vi "PicoScope6000aExampleRapidBlockBulk.vi"() -> ()   [LabVIEW 2009]
uses:
  <vilib>/Waveform/DWDTOps.llb/DWDT Analog to Digital.vi
panel:
  in  "Channels":T1 {"Channel H Settings"."Range" items=["10mV", "20mV", "50mV", "100mV", "200mV", "500mV", "1V", "2V", "5V", "10V", "20V", "50V", "100V", "200V", "x10_Probe_100mV", "x10_Probe_200mV", "x10_Probe_500mV", "x10_Probe_1V", "x10_Probe_2V", "x10_Probe_5V", "x10_Probe_10V", "x10_Probe_20V", "x10_Probe_50V", "x10_Probe_100V", "x10_Probe_200V", "x10_Probe_500V", "CURRENT_CLAMP_60A_2A", "CURRENT_CLAMP_60A_5A", "CURRENT_CLAMP_60A_10A", "CURRENT_CLAMP_60A_20A", "CURRENT_CLAMP_60A_50A", "CURRENT_CLAMP_60A_60A", "CURRENT_CLAMP_60A_V2_0_5A", "CURRENT_CLAMP_60A_V2_1A", "CURRENT_CLAMP_60A_V2_2A", "CURRENT_CLAMP_60A_V2_5A", "CURRENT_CLAMP_60A_V2_10A", "CURRENT_CLAMP_60A_V2_20A", "CURRENT_CLAMP_60A_V2_50A", "CURRENT_CLAMP_60A_V2_60A", "RESISTANCE_LEAD_NEG5_TO_20OHM", "RESISTANCE_LEAD_NEG50_TO_200OHM", "RESISTANCE_LEAD_NEG500_TO_2KOHM", "RESISTANCE_LEAD_NEG5K_TO_20KOHM", "RESISTANCE_LEAD_NEG50K_TO_LEAD_200KOHM", "RESISTANCE_LEAD_NEG500K_TO_LEAD_2MOHM", "RESISTANCE_LEAD_DIODE_TEST", "HT_NEG3_TO_5KV", "HT_NEG3_TO_10KV", "HT_NEG5_TO_20KV", "HT_NEG5_TO_50KV", "HT_NEG5_TO_100KV", "HT_NEG3_TO_5KV_INVERTED", "HT_NEG3_TO_10KV_INVERTED", "HT_NEG5_TO_20KV_INVERTED", "HT_NEG5_TO_50KV_INVERTED", "HT_NEG5_TO_100KV_INVERTED", "TEMPERATURE_NEG50_TO_150DEGC", "PRESSURE_SENSOR_-100k-150k_PASCALS", "PRESSURE_SENSOR_-100k_TO_400k_PASCALS", "PRESSURE_SENSOR_-200k_TO_800k_PASCALS", "PRESSURE_SENSOR_-400k_TO_1600k_PASCALS", "PRESSURE_SENSOR_-400k_TO_3400k_PASCALS", "PRESSURE_SENSOR_-150k_TO_1350k_PASCALS"]; "Channel H Settings"."BandWidth" items=["Full", "100kHz", "20kHz", "1MHz", "20MHz", "25MHz", "50MHz", "250MHz", "500MHz"]; "Channel H Settings"."Coupling" items=["AC", "DC"]; "Channel G Settings"."Range" items=["10mV", "20mV", "50mV", "100mV", "200mV", "500mV", "1V", "2V", "5V", "10V", "20V", "50V", "100V", "200V", "x10_Probe_100mV", "x10_Probe_200mV", "x10_Probe_500mV", "x10_Probe_1V", "x10_Probe_2V", "x10_Probe_5V", "x10_Probe_10V", "x10_Probe_20V", "x10_Probe_50V", "x10_Probe_100V", "x10_Probe_200V", "x10_Probe_500V", "CURRENT_CLAMP_60A_2A", "CURRENT_CLAMP_60A_5A", "CURRENT_CLAMP_60A_10A", "CURRENT_CLAMP_60A_20A", "CURRENT_CLAMP_60A_50A", "CURRENT_CLAMP_60A_60A", "CURRENT_CLAMP_60A_V2_0_5A", "CURRENT_CLAMP_60A_V2_1A", "CURRENT_CLAMP_60A_V2_2A", "CURRENT_CLAMP_60A_V2_5A", "CURRENT_CLAMP_60A_V2_10A", "CURRENT_CLAMP_60A_V2_20A", "CURRENT_CLAMP_60A_V2_50A", "CURRENT_CLAMP_60A_V2_60A", "RESISTANCE_LEAD_NEG5_TO_20OHM", "RESISTANCE_LEAD_NEG50_TO_200OHM", "RESISTANCE_LEAD_NEG500_TO_2KOHM", "RESISTANCE_LEAD_NEG5K_TO_20KOHM", "RESISTANCE_LEAD_NEG50K_TO_LEAD_200KOHM", "RESISTANCE_LEAD_NEG500K_TO_LEAD_2MOHM", "RESISTANCE_LEAD_DIODE_TEST", "HT_NEG3_TO_5KV", "HT_NEG3_TO_10KV", "HT_NEG5_TO_20KV", "HT_NEG5_TO_50KV", "HT_NEG5_TO_100KV", "HT_NEG3_TO_5KV_INVERTED", "HT_NEG3_TO_10KV_INVERTED", "HT_NEG5_TO_20KV_INVERTED", "HT_NEG5_TO_50KV_INVERTED", "HT_NEG5_TO_100KV_INVERTED", "TEMPERATURE_NEG50_TO_150DEGC", "PRESSURE_SENSOR_-100k-150k_PASCALS", "PRESSURE_SENSOR_-100k_TO_400k_PASCALS", "PRESSURE_SENSOR_-200k_TO_800k_PASCALS", "PRESSURE_SENSOR_-400k_TO_1600k_PASCALS", "PRESSURE_SENSOR_-400k_TO_3400k_PASCALS", "PRESSURE_SENSOR_-150k_TO_1350k_PASCALS"]; "Channel G Settings"."BandWidth" items=["Full", "100kHz", "20kHz", "1MHz", "20MHz", "25MHz", "50MHz", "250MHz", "500MHz"]; "Channel G Settings"."Coupling" items=["AC", "DC"]; "Channel F Settings"."Range" items=["10mV", "20mV", "50mV", "100mV", "200mV", "500mV", "1V", "2V", "5V", "10V", "20V", "50V", "100V", "200V", "x10_Probe_100mV", "x10_Probe_200mV", "x10_Probe_500mV", "x10_Probe_1V", "x10_Probe_2V", "x10_Probe_5V", "x10_Probe_10V", "x10_Probe_20V", "x10_Probe_50V", "x10_Probe_100V", "x10_Probe_200V", "x10_Probe_500V", "CURRENT_CLAMP_60A_2A", "CURRENT_CLAMP_60A_5A", "CURRENT_CLAMP_60A_10A", "CURRENT_CLAMP_60A_20A", "CURRENT_CLAMP_60A_50A", "CURRENT_CLAMP_60A_60A", "CURRENT_CLAMP_60A_V2_0_5A", "CURRENT_CLAMP_60A_V2_1A", "CURRENT_CLAMP_60A_V2_2A", "CURRENT_CLAMP_60A_V2_5A", "CURRENT_CLAMP_60A_V2_10A", "CURRENT_CLAMP_60A_V2_20A", "CURRENT_CLAMP_60A_V2_50A", "CURRENT_CLAMP_60A_V2_60A", "RESISTANCE_LEAD_NEG5_TO_20OHM", "RESISTANCE_LEAD_NEG50_TO_200OHM", "RESISTANCE_LEAD_NEG500_TO_2KOHM", "RESISTANCE_LEAD_NEG5K_TO_20KOHM", "RESISTANCE_LEAD_NEG50K_TO_LEAD_200KOHM", "RESISTANCE_LEAD_NEG500K_TO_LEAD_2MOHM", "RESISTANCE_LEAD_DIODE_TEST", "HT_NEG3_TO_5KV", "HT_NEG3_TO_10KV", "HT_NEG5_TO_20KV", "HT_NEG5_TO_50KV", "HT_NEG5_TO_100KV", "HT_NEG3_TO_5KV_INVERTED", "HT_NEG3_TO_10KV_INVERTED", "HT_NEG5_TO_20KV_INVERTED", "HT_NEG5_TO_50KV_INVERTED", "HT_NEG5_TO_100KV_INVERTED", "TEMPERATURE_NEG50_TO_150DEGC", "PRESSURE_SENSOR_-100k-150k_PASCALS", "PRESSURE_SENSOR_-100k_TO_400k_PASCALS", "PRESSURE_SENSOR_-200k_TO_800k_PASCALS", "PRESSURE_SENSOR_-400k_TO_1600k_PASCALS", "PRESSURE_SENSOR_-400k_TO_3400k_PASCALS", "PRESSURE_SENSOR_-150k_TO_1350k_PASCALS"]; "Channel F Settings"."BandWidth" items=["Full", "100kHz", "20kHz", "1MHz", "20MHz", "25MHz", "50MHz", "250MHz", "500MHz"]; "Channel F Settings"."Coupling" items=["AC", "DC"]; "Channel E Settings"."Range" items=["10mV", "20mV", "50mV", "100mV", "200mV", "500mV", "1V", "2V", "5V", "10V", "20V", "50V", "100V", "200V", "x10_Probe_100mV", "x10_Probe_200mV", "x10_Probe_500mV", "x10_Probe_1V", "x10_Probe_2V", "x10_Probe_5V", "x10_Probe_10V", "x10_Probe_20V", "x10_Probe_50V", "x10_Probe_100V", "x10_Probe_200V", "x10_Probe_500V", "CURRENT_CLAMP_60A_2A", "CURRENT_CLAMP_60A_5A", "CURRENT_CLAMP_60A_10A", "CURRENT_CLAMP_60A_20A", "CURRENT_CLAMP_60A_50A", "CURRENT_CLAMP_60A_60A", "CURRENT_CLAMP_60A_V2_0_5A", "CURRENT_CLAMP_60A_V2_1A", "CURRENT_CLAMP_60A_V2_2A", "CURRENT_CLAMP_60A_V2_5A", "CURRENT_CLAMP_60A_V2_10A", "CURRENT_CLAMP_60A_V2_20A", "CURRENT_CLAMP_60A_V2_50A", "CURRENT_CLAMP_60A_V2_60A", "RESISTANCE_LEAD_NEG5_TO_20OHM", "RESISTANCE_LEAD_NEG50_TO_200OHM", "RESISTANCE_LEAD_NEG500_TO_2KOHM", "RESISTANCE_LEAD_NEG5K_TO_20KOHM", "RESISTANCE_LEAD_NEG50K_TO_LEAD_200KOHM", "RESISTANCE_LEAD_NEG500K_TO_LEAD_2MOHM", "RESISTANCE_LEAD_DIODE_TEST", "HT_NEG3_TO_5KV", "HT_NEG3_TO_10KV", "HT_NEG5_TO_20KV", "HT_NEG5_TO_50KV", "HT_NEG5_TO_100KV", "HT_NEG3_TO_5KV_INVERTED", "HT_NEG3_TO_10KV_INVERTED", "HT_NEG5_TO_20KV_INVERTED", "HT_NEG5_TO_50KV_INVERTED", "HT_NEG5_TO_100KV_INVERTED", "TEMPERATURE_NEG50_TO_150DEGC", "PRESSURE_SENSOR_-100k-150k_PASCALS", "PRESSURE_SENSOR_-100k_TO_400k_PASCALS", "PRESSURE_SENSOR_-200k_TO_800k_PASCALS", "PRESSURE_SENSOR_-400k_TO_1600k_PASCALS", "PRESSURE_SENSOR_-400k_TO_3400k_PASCALS", "PRESSURE_SENSOR_-150k_TO_1350k_PASCALS"]; "Channel E Settings"."BandWidth" items=["Full", "100kHz", "20kHz", "1MHz", "20MHz", "25MHz", "50MHz", "250MHz", "500MHz"]; "Channel E Settings"."Coupling" items=["AC", "DC"]; "Channel D Settings"."Range" items=["10mV", "20mV", "50mV", "100mV", "200mV", "500mV", "1V", "2V", "5V", "10V", "20V", "50V", "100V", "200V", "x10_Probe_100mV", "x10_Probe_200mV", "x10_Probe_500mV", "x10_Probe_1V", "x10_Probe_2V", "x10_Probe_5V", "x10_Probe_10V", "x10_Probe_20V", "x10_Probe_50V", "x10_Probe_100V", "x10_Probe_200V", "x10_Probe_500V", "CURRENT_CLAMP_60A_2A", "CURRENT_CLAMP_60A_5A", "CURRENT_CLAMP_60A_10A", "CURRENT_CLAMP_60A_20A", "CURRENT_CLAMP_60A_50A", "CURRENT_CLAMP_60A_60A", "CURRENT_CLAMP_60A_V2_0_5A", "CURRENT_CLAMP_60A_V2_1A", "CURRENT_CLAMP_60A_V2_2A", "CURRENT_CLAMP_60A_V2_5A", "CURRENT_CLAMP_60A_V2_10A", "CURRENT_CLAMP_60A_V2_20A", "CURRENT_CLAMP_60A_V2_50A", "CURRENT_CLAMP_60A_V2_60A", "RESISTANCE_LEAD_NEG5_TO_20OHM", "RESISTANCE_LEAD_NEG50_TO_200OHM", "RESISTANCE_LEAD_NEG500_TO_2KOHM", "RESISTANCE_LEAD_NEG5K_TO_20KOHM", "RESISTANCE_LEAD_NEG50K_TO_LEAD_200KOHM", "RESISTANCE_LEAD_NEG500K_TO_LEAD_2MOHM", "RESISTANCE_LEAD_DIODE_TEST", "HT_NEG3_TO_5KV", "HT_NEG3_TO_10KV", "HT_NEG5_TO_20KV", "HT_NEG5_TO_50KV", "HT_NEG5_TO_100KV", "HT_NEG3_TO_5KV_INVERTED", "HT_NEG3_TO_10KV_INVERTED", "HT_NEG5_TO_20KV_INVERTED", "HT_NEG5_TO_50KV_INVERTED", "HT_NEG5_TO_100KV_INVERTED", "TEMPERATURE_NEG50_TO_150DEGC", "PRESSURE_SENSOR_-100k-150k_PASCALS", "PRESSURE_SENSOR_-100k_TO_400k_PASCALS", "PRESSURE_SENSOR_-200k_TO_800k_PASCALS", "PRESSURE_SENSOR_-400k_TO_1600k_PASCALS", "PRESSURE_SENSOR_-400k_TO_3400k_PASCALS", "PRESSURE_SENSOR_-150k_TO_1350k_PASCALS"]; "Channel D Settings"."BandWidth" items=["Full", "100kHz", "20kHz", "1MHz", "20MHz", "25MHz", "50MHz", "250MHz", "500MHz"]; "Channel D Settings"."Coupling" items=["AC", "DC"]; "Channel C Settings"."Range" items=["10mV", "20mV", "50mV", "100mV", "200mV", "500mV", "1V", "2V", "5V", "10V", "20V", "50V", "100V", "200V", "x10_Probe_100mV", "x10_Probe_200mV", "x10_Probe_500mV", "x10_Probe_1V", "x10_Probe_2V", "x10_Probe_5V", "x10_Probe_10V", "x10_Probe_20V", "x10_Probe_50V", "x10_Probe_100V", "x10_Probe_200V", "x10_Probe_500V", "CURRENT_CLAMP_60A_2A", "CURRENT_CLAMP_60A_5A", "CURRENT_CLAMP_60A_10A", "CURRENT_CLAMP_60A_20A", "CURRENT_CLAMP_60A_50A", "CURRENT_CLAMP_60A_60A", "CURRENT_CLAMP_60A_V2_0_5A", "CURRENT_CLAMP_60A_V2_1A", "CURRENT_CLAMP_60A_V2_2A", "CURRENT_CLAMP_60A_V2_5A", "CURRENT_CLAMP_60A_V2_10A", "CURRENT_CLAMP_60A_V2_20A", "CURRENT_CLAMP_60A_V2_50A", "CURRENT_CLAMP_60A_V2_60A", "RESISTANCE_LEAD_NEG5_TO_20OHM", "RESISTANCE_LEAD_NEG50_TO_200OHM", "RESISTANCE_LEAD_NEG500_TO_2KOHM", "RESISTANCE_LEAD_NEG5K_TO_20KOHM", "RESISTANCE_LEAD_NEG50K_TO_LEAD_200KOHM", "RESISTANCE_LEAD_NEG500K_TO_LEAD_2MOHM", "RESISTANCE_LEAD_DIODE_TEST", "HT_NEG3_TO_5KV", "HT_NEG3_TO_10KV", "HT_NEG5_TO_20KV", "HT_NEG5_TO_50KV", "HT_NEG5_TO_100KV", "HT_NEG3_TO_5KV_INVERTED", "HT_NEG3_TO_10KV_INVERTED", "HT_NEG5_TO_20KV_INVERTED", "HT_NEG5_TO_50KV_INVERTED", "HT_NEG5_TO_100KV_INVERTED", "TEMPERATURE_NEG50_TO_150DEGC", "PRESSURE_SENSOR_-100k-150k_PASCALS", "PRESSURE_SENSOR_-100k_TO_400k_PASCALS", "PRESSURE_SENSOR_-200k_TO_800k_PASCALS", "PRESSURE_SENSOR_-400k_TO_1600k_PASCALS", "PRESSURE_SENSOR_-400k_TO_3400k_PASCALS", "PRESSURE_SENSOR_-150k_TO_1350k_PASCALS"]; "Channel C Settings"."BandWidth" items=["Full", "100kHz", "20kHz", "1MHz", "20MHz", "25MHz", "50MHz", "250MHz", "500MHz"]; "Channel C Settings"."Coupling" items=["AC", "DC"]; "Channel B Settings"."Range" items=["10mV", "20mV", "50mV", "100mV", "200mV", "500mV", "1V", "2V", "5V", "10V", "20V", "50V", "100V", "200V", "x10_Probe_100mV", "x10_Probe_200mV", "x10_Probe_500mV", "x10_Probe_1V", "x10_Probe_2V", "x10_Probe_5V", "x10_Probe_10V", "x10_Probe_20V", "x10_Probe_50V", "x10_Probe_100V", "x10_Probe_200V", "x10_Probe_500V", "CURRENT_CLAMP_60A_2A", "CURRENT_CLAMP_60A_5A", "CURRENT_CLAMP_60A_10A", "CURRENT_CLAMP_60A_20A", "CURRENT_CLAMP_60A_50A", "CURRENT_CLAMP_60A_60A", "CURRENT_CLAMP_60A_V2_0_5A", "CURRENT_CLAMP_60A_V2_1A", "CURRENT_CLAMP_60A_V2_2A", "CURRENT_CLAMP_60A_V2_5A", "CURRENT_CLAMP_60A_V2_10A", "CURRENT_CLAMP_60A_V2_20A", "CURRENT_CLAMP_60A_V2_50A", "CURRENT_CLAMP_60A_V2_60A", "RESISTANCE_LEAD_NEG5_TO_20OHM", "RESISTANCE_LEAD_NEG50_TO_200OHM", "RESISTANCE_LEAD_NEG500_TO_2KOHM", "RESISTANCE_LEAD_NEG5K_TO_20KOHM", "RESISTANCE_LEAD_NEG50K_TO_LEAD_200KOHM", "RESISTANCE_LEAD_NEG500K_TO_LEAD_2MOHM", "RESISTANCE_LEAD_DIODE_TEST", "HT_NEG3_TO_5KV", "HT_NEG3_TO_10KV", "HT_NEG5_TO_20KV", "HT_NEG5_TO_50KV", "HT_NEG5_TO_100KV", "HT_NEG3_TO_5KV_INVERTED", "HT_NEG3_TO_10KV_INVERTED", "HT_NEG5_TO_20KV_INVERTED", "HT_NEG5_TO_50KV_INVERTED", "HT_NEG5_TO_100KV_INVERTED", "TEMPERATURE_NEG50_TO_150DEGC", "PRESSURE_SENSOR_-100k-150k_PASCALS", "PRESSURE_SENSOR_-100k_TO_400k_PASCALS", "PRESSURE_SENSOR_-200k_TO_800k_PASCALS", "PRESSURE_SENSOR_-400k_TO_1600k_PASCALS", "PRESSURE_SENSOR_-400k_TO_3400k_PASCALS", "PRESSURE_SENSOR_-150k_TO_1350k_PASCALS"]; "Channel B Settings"."BandWidth" items=["Full", "100kHz", "20kHz", "1MHz", "20MHz", "25MHz", "50MHz", "250MHz", "500MHz"]; "Channel B Settings"."Coupling" items=["AC", "DC"]; "Channel A Settings"."Range" items=["10mV", "20mV", "50mV", "100mV", "200mV", "500mV", "1V", "2V", "5V", "10V", "20V", "50V", "100V", "200V", "x10_Probe_100mV", "x10_Probe_200mV", "x10_Probe_500mV", "x10_Probe_1V", "x10_Probe_2V", "x10_Probe_5V", "x10_Probe_10V", "x10_Probe_20V", "x10_Probe_50V", "x10_Probe_100V", "x10_Probe_200V", "x10_Probe_500V", "CURRENT_CLAMP_60A_2A", "CURRENT_CLAMP_60A_5A", "CURRENT_CLAMP_60A_10A", "CURRENT_CLAMP_60A_20A", "CURRENT_CLAMP_60A_50A", "CURRENT_CLAMP_60A_60A", "CURRENT_CLAMP_60A_V2_0_5A", "CURRENT_CLAMP_60A_V2_1A", "CURRENT_CLAMP_60A_V2_2A", "CURRENT_CLAMP_60A_V2_5A", "CURRENT_CLAMP_60A_V2_10A", "CURRENT_CLAMP_60A_V2_20A", "CURRENT_CLAMP_60A_V2_50A", "CURRENT_CLAMP_60A_V2_60A", "RESISTANCE_LEAD_NEG5_TO_20OHM", "RESISTANCE_LEAD_NEG50_TO_200OHM", "RESISTANCE_LEAD_NEG500_TO_2KOHM", "RESISTANCE_LEAD_NEG5K_TO_20KOHM", "RESISTANCE_LEAD_NEG50K_TO_LEAD_200KOHM", "RESISTANCE_LEAD_NEG500K_TO_LEAD_2MOHM", "RESISTANCE_LEAD_DIODE_TEST", "HT_NEG3_TO_5KV", "HT_NEG3_TO_10KV", "HT_NEG5_TO_20KV", "HT_NEG5_TO_50KV", "HT_NEG5_TO_100KV", "HT_NEG3_TO_5KV_INVERTED", "HT_NEG3_TO_10KV_INVERTED", "HT_NEG5_TO_20KV_INVERTED", "HT_NEG5_TO_50KV_INVERTED", "HT_NEG5_TO_100KV_INVERTED", "TEMPERATURE_NEG50_TO_150DEGC", "PRESSURE_SENSOR_-100k-150k_PASCALS", "PRESSURE_SENSOR_-100k_TO_400k_PASCALS", "PRESSURE_SENSOR_-200k_TO_800k_PASCALS", "PRESSURE_SENSOR_-400k_TO_1600k_PASCALS", "PRESSURE_SENSOR_-400k_TO_3400k_PASCALS", "PRESSURE_SENSOR_-150k_TO_1350k_PASCALS"]; "Channel A Settings"."BandWidth" items=["Full", "100kHz", "20kHz", "1MHz", "20MHz", "25MHz", "50MHz", "250MHz", "500MHz"]; "Channel A Settings"."Coupling" items=["AC", "DC"]}
  out "overflow":i16[](array[numeric]) format="%08b"
  out "nMaxSamples":u64
  in  "Buffer and Transfer Settings":T2 {"Down-Sample Mode" items=["None", "Aggregate", "Decimate", "Average"]; "Down Sample Ratio" step=1; "noOfSamples" format="%#_6p"}
  in  "Acquisition Settings":T3 {"postTriggerSamples" format="%#_6p"; "preTriggerSamples" format="%#_6p"}
  out "Capture Complete":bool
  out "Number of Samples \nPer Capture":u64 format="%#_6p"
  in  "Run":bool
  in  "Capture Index":i16 min=0
  in  "Digital Channels":T4 {"Port 1 Settings"."Hysteresis" items=["PICO_VERY_HIGH_400MV", "PICO_HIGH_200MV", "PICO_NORMAL_100MV", "PICO_LOW_50MV"]; "Port 0 Settings"."Hysteresis" items=["PICO_VERY_HIGH_400MV", "PICO_HIGH_200MV", "PICO_NORMAL_100MV", "PICO_LOW_50MV"]}
  out "Properties Panel":T5 {"Max Total Capture Time Available (sec)" format="%.3p"; "Sample Frequency" format="%.6p"; "Sample Rate" format="%.3p"; "Max Samples Available" format="%_6p"; "Total Capture Time (sec)" format="%.3p"}
  out "Port 0":digitalwaveform(graph)
  in  "Trigger Settings":T6 {"Trigger Source" items=["Channel A", "Channel B", "Channel C", "Channel D", "Channel E", "Channel F", "Channel G", "Channel H", "Port 0", "Port 1", "Trigger AUX"]; "Trigger Direction" items=["Rising", "Falling"]; "Trigger Threshold (Volts)" format="%#_6p"}
  in  "stop":bool
  out "Analog Channels":cluster{i32, dbl, "Data (Volts)":dbl[]}[](graph)
  out "Device Info":T7
  out "Pico 6000a Units":string
  in  "Resolution":u32(ring) items=["8-bit", "12-bit", "14-bit", "15-bit", "16-bit", "10-bit"]
  in  "Serial Number":string
  in  "Use Serial Number":bool
  in  "error in (no error)":errorcluster
  # "Please Ensure you set the \"Range\"(Probe type) before running the VI"
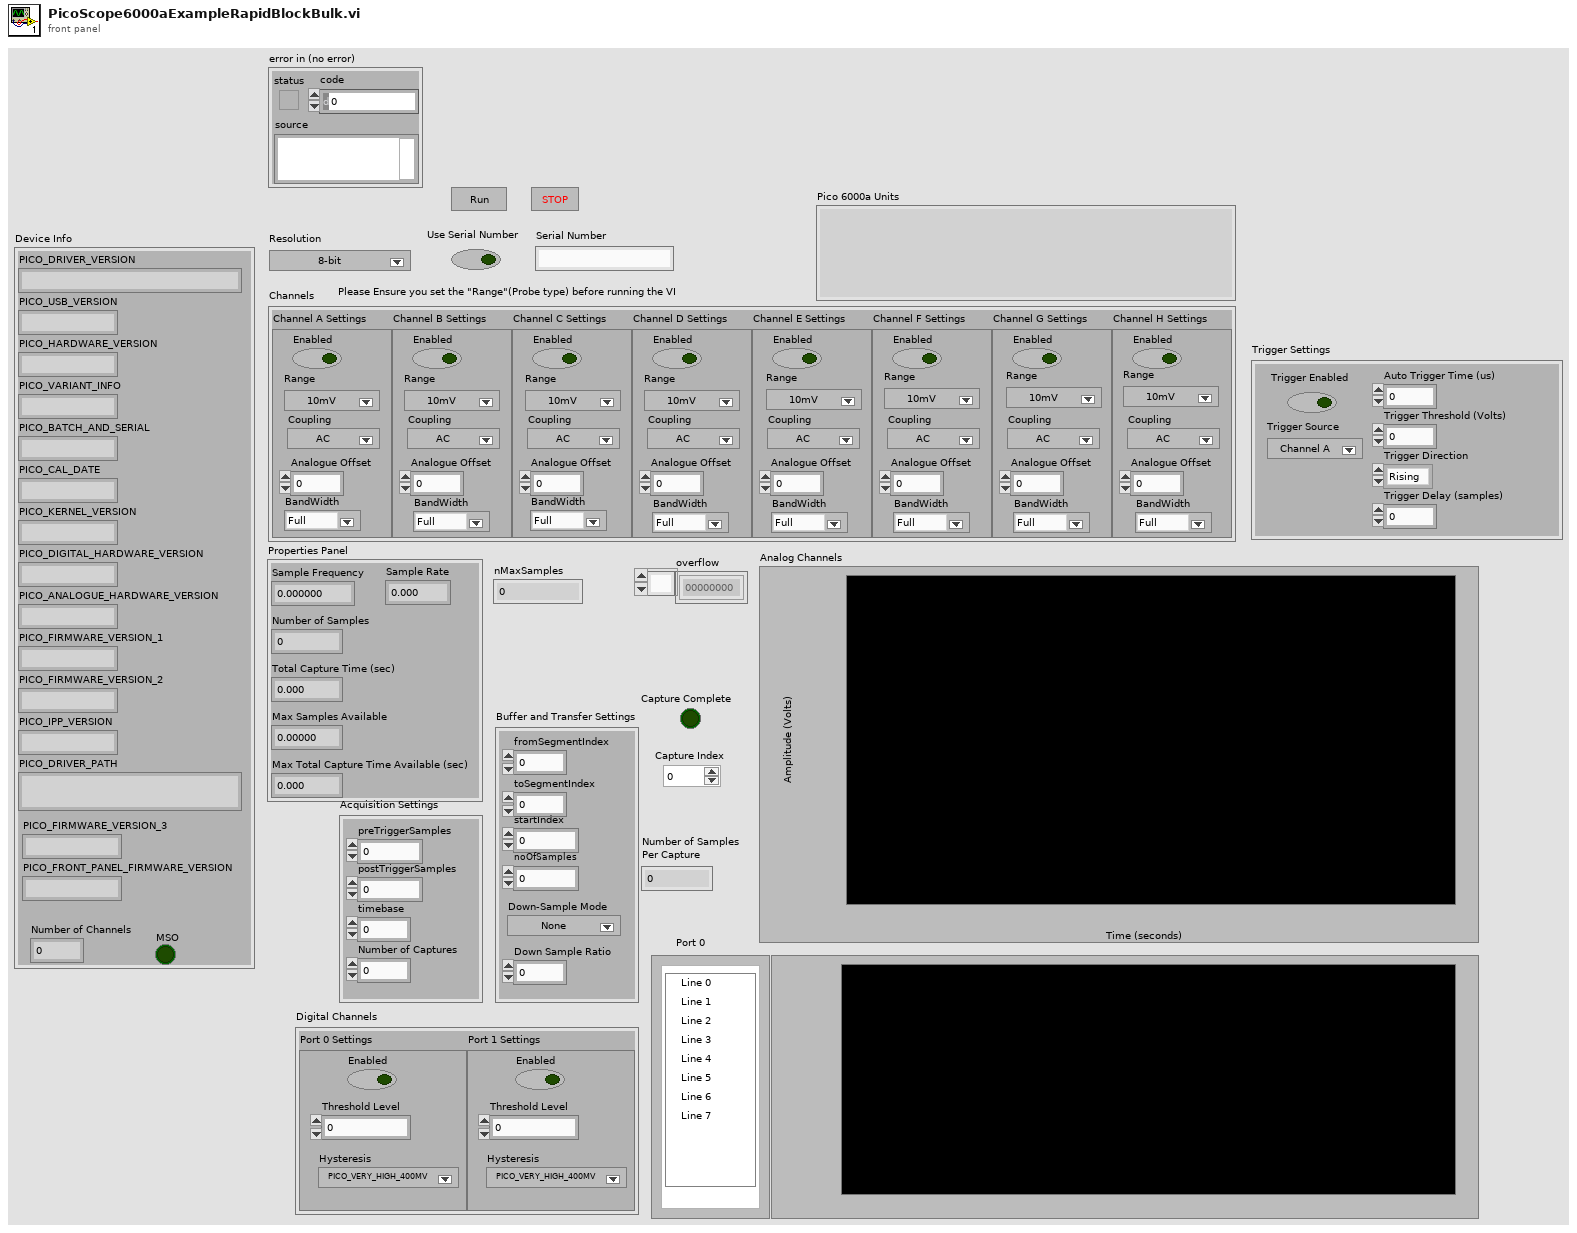
[diagram p1: front panel]
types:
  T1 = cluster{"Channel A Settings ":cluster{"Enabled":bool, "Coupling":i16, "Range":u16, "Analogue Offset":dbl, "BandWidth":u32}, "Channel B Settings ":cluster{"Enabled":bool, "Coupling":i16, "Range":u16, "Analogue Offset":dbl, "BandWidth":u32}, "Channel C Settings ":cluster{"Enabled":bool, "Coupling":i16, "Range":u16, "Analogue Offset":dbl, "BandWidth":u32}, "Channel D Settings ":cluster{"Enabled":bool, "Coupling":i16, "Range":u16, "Analogue Offset":dbl, "BandWidth":u32}, "Channel E Settings":cluster{"Enabled":bool, "Coupling":i16, "Range":u16, "Analogue Offset":dbl, "BandWidth":u32}, "Channel F Settings":cluster{"Enabled":bool, "Coupling":i16, "Range":u16, "Analogue Offset":dbl, "BandWidth":u32}, "Channel G Settings":cluster{"Enabled":bool, "Coupling":i16, "Range":u16, "Analogue Offset":dbl, "BandWidth":u32}, "Channel H Settings ":cluster{"Enabled":bool, "Coupling":i16, "Range":u16, "Analogue Offset":dbl, "BandWidth":u32}}
  T2 = cluster{"fromSegmentIndex":u64, "toSegmentIndex":u64, "startIndex":u64, "noOfSamples":u64, "Down-Sample Mode":u32, "Down Sample Ratio":u64}
  T3 = cluster{"preTriggerSamples":u64, "postTriggerSamples":u64, "timebase":u32, "Number of Captures":u64}
  T4 = cluster{"Port 0 Settings ":cluster{"Enabled":bool, "Threshold Level":i16, "Hysteresis":u32}, "Port 1 Settings":cluster{"Enabled":bool, "Threshold Level":i16, "Hysteresis":u32}}
  T5 = cluster{"Sample Frequency":dbl, "Sample Rate":dbl, "Max Samples Available":u64, "Number of Samples":u64, "Total Capture Time (sec) ":dbl, "Max Total Capture Time Available (sec)":dbl}
  T6 = cluster{"Trigger Enabled":bool, "Trigger Threshold (Volts)":dbl, "Trigger Direction":u16, "Trigger Delay (samples)":u64, "Auto Trigger Time (us)":u32, "Trigger Source":u32}
  T7 = cluster{"PICO_DRIVER_VERSION":string, "PICO_USB_VERSION":string, "PICO_HARDWARE_VERSION":string, "PICO_VARIANT_INFO":string, "PICO_BATCH_AND_SERIAL":string, "PICO_CAL_DATE":string, "PICO_KERNEL_VERSION":string, "PICO_DIGITAL_HARDWARE_VERSION":string, "PICO_ANALOGUE_HARDWARE_VERSION":string, "PICO_FIRMWARE_VERSION_1":string, "PICO_FIRMWARE_VERSION_2":string, "PICO_IPP_VERSION":string, "PICO_DRIVER_PATH":string, "PICO_FIRMWARE_VERSION_3":string, "PICO_FRONT_PANEL_FIRMWARE_VERSION":string, "Number of Channels":i16, "MSO":bool}
  T8 = cluster{"bufferMax ChA":i16[][], "bufferMax ChB":i16[][], "bufferMax ChC":i16[][], "bufferMax ChD":i16[][], "bufferMax ChE":i16[][], "bufferMin ChF":i16[][], "bufferMin ChG":i16[][], "bufferMax ChH":i16[][], "bufferMax Port0":i16[][], "bufferMax Port1":i16[][]}
  T9 = cluster{"preTriggerSamples":u64, "postTriggerSamples":u64, "timebase":u32}
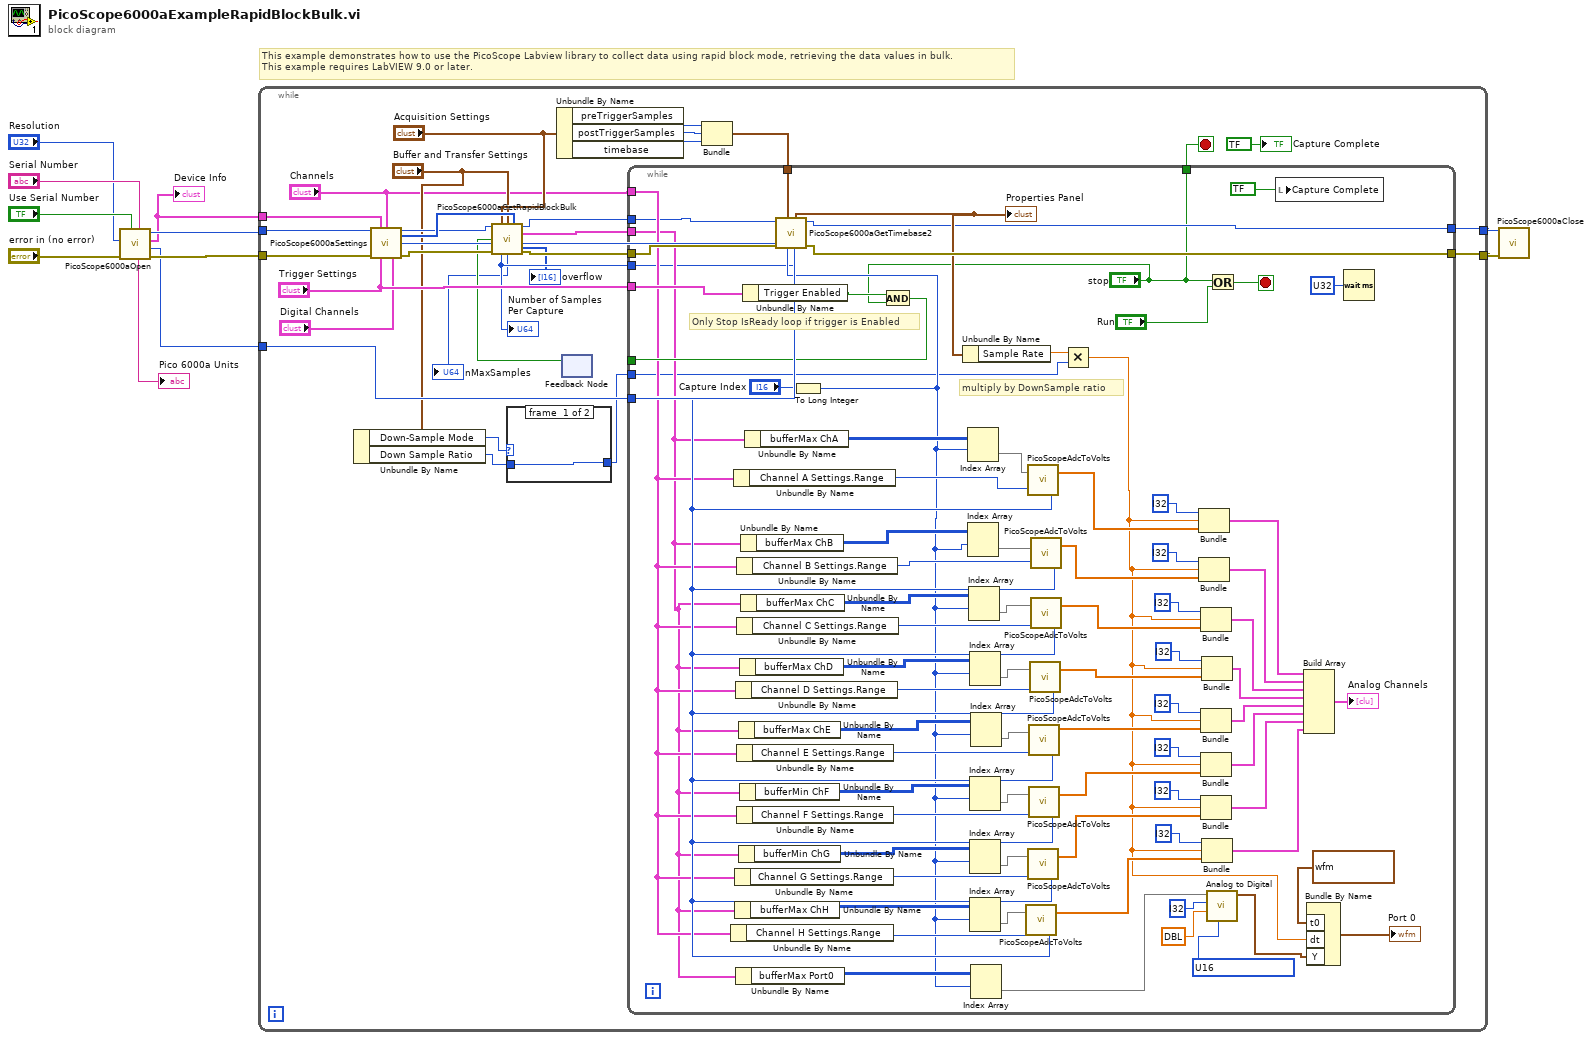
[diagram p0: block diagram]
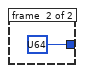
[diagram p2: hidden frame]
diagram:
  # "This example demonstrates how to use the PicoScope Labview library to collect data using rapid block mode, retrieving the data values in bulk.\nThis example requires LabVIEW 9.0 or later."
  n1 = call "PicoScope6000aOpen.vi"("Serial Number"="Serial Number", "Use Serial Number"="Use Serial Number", "error in (no error)"="error in (no error)", "Resolution"="Resolution") -> ("error out"=w7:errorcluster, "Max ADC value"=w1:i16, "Device Info"=w2:T7, "handle out"=w8:i16, "Pico 6000a Units"=→"Pico 6000a Units":string)  [unwired: 2 in, 1 out]
  "Device Info" <- w2
  n2 = while {
    tunnel: w2 -> [w40]
    tunnel: w1 -> [w37]
    tunnel: w8 -> [w42]
    tunnel: [w34] -> w6
    tunnel: w7 -> [w41]
    tunnel: [w35] -> w5
    stop <- w30 stop-if-true
    n3 = Unbundle By Name("Buffer and Transfer Settings") -> ("Down-Sample Mode"=w17:u32, "Down Sample Ratio"=w16:u64)
    n4 = call "PicoScope6000aSettings.vi"("handle in"=w42, "Device Info"=w40, "Channels"="Channels", "Max ADC value"=w37, "error in (no error)"=w41, "Trigger Settings"="Trigger Settings", "Digital Channels"="Digital Channels") -> ("Enabled array"=w39:i16[], "handle out"=w27:i16, "error out"=w29:errorcluster)  [unwired: 6 in]
    n5 = case shown="80000000" w17 {
      tunnel: [w43 u64 ? ("Down Sample Ratio")] -> w15
      tunnel: w16 -> [w43 _]
      frame #0 {
      }
      frame #1 {
      }
    }
    n6 = Unbundle By Name("Acquisition Settings") -> ("preTriggerSamples"=w23:u64, "postTriggerSamples"=w22:u64, "timebase"=w21:u32)
    n7 = feedback #1() -> (w24:bool)  [unwired: 1 in]
    n8 = call "PicoScope6000aGetRapidBlockBulk.vi"("handle in"=w27, "Acquisition Settings"="Acquisition Settings", "Buffer and Transfer Settings"="Buffer and Transfer Settings", "enabled array"=w39, "stop IsReady"=w24, "error in (no error)"=w29) -> ("handle out"=w26:i16, "Buffers (Max or non-aggregated)"=w33:T8, "noOfSamples"=w32:u64, "nMaxSamples"=→"nMaxSamples":u64, "overflow"=→"overflow":i16[], "error out"=w28:errorcluster)  [unwired: 3 in, 1 out]
    "Number of Samples \nPer Capture" <- w32
    n9 = Bundle("preTriggerSamples"=w23, "postTriggerSamples"=w22, "timebase"=w21) -> (w20:T9)  [unwired: 1 in]
    n10 = while {
      tunnel: "Trigger Settings" -> [w85]
      tunnel: w37 -> [w83]
      tunnel: [w82] -> w25
      tunnel: "Channels" -> [w72]
      tunnel: w33 -> [w62]
      tunnel: w32 -> [w60]
      tunnel: [w75] -> w34
      tunnel: w26 -> [w57]
      tunnel: w28 -> [w78]
      tunnel: [w77] -> w35
      tunnel: ["stop"] -> w30
      tunnel: w20 -> [w54]
      tunnel: w15 -> [w45]
      stop <- w56 stop-if-true
      w90 = u16 ? items=["unsigned binary", "offset binary", "2's complement"] ("data format (offset binary)")
      # "multiply by DownSample ratio"
      # "Only Stop IsReady loop if trigger is Enabled"
      n11 = Unbundle By Name(w72) -> ("Channel H Settings.Range"=w110:u16)
      n12 = Unbundle By Name(w72) -> ("Channel A Settings.Range"=w123:u16)
      n13 = Unbundle By Name(w72) -> ("Channel G Settings.Range"=w111:u16)
      n14 = Unbundle By Name(w62) -> ("bufferMax ChH"=w69:i16[][])
      n15 = Unbundle By Name(w72) -> ("Channel D Settings.Range"=w114:u16)
      n16 = Unbundle By Name(w62) -> ("bufferMax Port0"=w73:i16[][])
      n17 = Unbundle By Name(w72) -> ("Channel B Settings.Range"=w121:u16)
      n18 = Unbundle By Name(w72) -> ("Channel C Settings.Range"=w115:u16)
      n19 = Unbundle By Name(w72) -> ("Channel E Settings.Range"=w113:u16)
      n20 = Unbundle By Name(w72) -> ("Channel F Settings.Range"=w112:u16)
      n21 = Unbundle By Name(w62) -> ("bufferMax ChE"=w66:i16[][])
      n22 = Unbundle By Name(w62) -> ("bufferMin ChG"=w68:i16[][])
      n23 = Unbundle By Name(w62) -> ("bufferMax ChD"=w65:i16[][])
      n24 = Unbundle By Name(w62) -> ("bufferMin ChF"=w67:i16[][])
      n25 = Unbundle By Name(w62) -> ("bufferMax ChB"=w70:i16[][])
      n26 = Unbundle By Name(w62) -> ("bufferMax ChC"=w64:i16[][])
      n27 = Unbundle By Name(w85) -> ("Trigger Enabled"=w84:bool)
      n28 = Unbundle By Name(w62) -> ("bufferMax ChA"=w80:i16[][])
      n29 = To Long Integer(number="Capture Index") -> (32bit integer=w63:i32)
      n30 = call "PicoScope6000aGetTimebase2.vi"("Number of Samples"=w60, "Memory Segment"=w63, "Acquisition Settings"=w54, "error in (no error)"=w78, "handle in"=w57) -> ("error out"=w77:errorcluster, "handle out"=w75:i16, "Properties Panel"=w76:T5)  [unwired: 4 in]
      "Properties Panel" <- w76
      n31 = And(x=w84, y="stop") -> (x .and. y?=w82:bool)
      n32 = Unbundle By Name(w76) -> ("Sample Rate"=w46:dbl)
      n33 = Index Array(array=w80, index (row)=w63) -> (element=w79:i16[])  [unwired: 1 in]
      n34 = Index Array(array=w70, index (row)=w63) -> (element=w71:i16[])  [unwired: 1 in]
      n35 = Index Array(array=w64, index (row)=w63) -> (element=w53:i16[])  [unwired: 1 in]
      n36 = Index Array(array=w65, index (row)=w63) -> (element=w52:i16[])  [unwired: 1 in]
      n37 = Index Array(array=w67, index (row)=w63) -> (element=w50:i16[])  [unwired: 1 in]
      n38 = Index Array(array=w68, index (row)=w63) -> (element=w49:i16[])  [unwired: 1 in]
      n39 = Index Array(array=w69, index (row)=w63) -> (element=w48:i16[])  [unwired: 1 in]
      n40 = Index Array(array=w66, index (row)=w63) -> (element=w51:i16[])  [unwired: 1 in]
      n41 = Index Array(array=w73, index (row)=w63) -> (element=w74:i16[])  [unwired: 1 in]
      n42 = call "PicoScopeAdcToVolts.vi"("Max_adc"=w83, "Range Index"=w110, "Data"=w48) -> ("Data (Volts)"=w105:dbl[])
      n43 = call "PicoScopeAdcToVolts.vi"("Max_adc"=w83, "Range Index"=w123, "Data"=w79) -> ("Data (Volts)"=w120:dbl[])
      n44 = call "PicoScopeAdcToVolts.vi"("Max_adc"=w83, "Range Index"=w111, "Data"=w49) -> ("Data (Volts)"=w99:dbl[])
      n45 = call "PicoScopeAdcToVolts.vi"("Max_adc"=w83, "Range Index"=w113, "Data"=w51) -> ("Data (Volts)"=w102:dbl[])
      n46 = call "PicoScopeAdcToVolts.vi"("Max_adc"=w83, "Range Index"=w112, "Data"=w50) -> ("Data (Volts)"=w98:dbl[])
      n47 = call "PicoScopeAdcToVolts.vi"("Max_adc"=w83, "Range Index"=w114, "Data"=w52) -> ("Data (Volts)"=w103:dbl[])
      n48 = call "PicoScopeAdcToVolts.vi"("Max_adc"=w83, "Range Index"=w121, "Data"=w71) -> ("Data (Volts)"=w119:dbl[])
      n49 = call "PicoScopeAdcToVolts.vi"("Max_adc"=w83, "Range Index"=w115, "Data"=w53) -> ("Data (Volts)"=w104:dbl[])
      n50 = Multiply(x=w46, y=w45) -> (x*y=w47:dbl)
      n51 = Bundle(i32 ?, w47, "Data (Volts)"=w120) -> (w118:cluster{i32, dbl, "Data (Volts)":dbl[]})  [unwired: 1 in]
      n52 = Bundle(i32 ?, w47, "Data (Volts)"=w119) -> (w117:cluster{i32, dbl, "Data (Volts)":dbl[]})  [unwired: 1 in]
      n53 = Bundle(i32 ?, w47, "Data (Volts)"=w104) -> (w97:cluster{i32, dbl, "Data (Volts)":dbl[]})  [unwired: 1 in]
      n54 = Bundle(i32 ?, w47, "Data (Volts)"=w102) -> (w95:cluster{i32, dbl, "Data (Volts)":dbl[]})  [unwired: 1 in]
      n55 = Bundle(i32 ?, w47, "Data (Volts)"=w98) -> (w94:cluster{i32, dbl, "Data (Volts)":dbl[]})  [unwired: 1 in]
      n56 = Bundle(i32 ?, w47, "Data (Volts)"=w99) -> (w93:cluster{i32, dbl, "Data (Volts)":dbl[]})  [unwired: 1 in]
      n57 = Bundle(i32 ?, w47, "Data (Volts)"=w103) -> (w96:cluster{i32, dbl, "Data (Volts)":dbl[]})  [unwired: 1 in]
      n58 = Bundle(i32 ?, w47, "Data (Volts)"=w105) -> (w92:cluster{i32, dbl, "Data (Volts)":dbl[]})  [unwired: 1 in]
      n59 = call-poly <vilib>:"Analog to Digital.vi"("data format (offset binary)"=w90, "full-scale range (pk-pk)"=dbl ?, "resolution (16 bit)"=i32 ?, "analog waveform"=w74) -> ("digital waveform"=w86:digitalwaveform)  [unwired: 4 in, 3 out]
      n60 = Or(x="stop", y="Run") -> (x .or. y?=w56:bool)
      n61 = local write "Capture Complete"(bool ? ("Capture Complete")) -> ()
      n62 = Build Array(w118, w117, w97, w96, w95, w94, w93, w92) -> (→"Analog Channels":cluster{i32, dbl, "Data (Volts)":dbl[]}[])
      n63 = Bundle By Name("t0"=timestamp ?, "dt"=w47, "Y"=w86) -> (→"Port 0":digitalwaveform)  [unwired: 1 in]
      n64 = Wait (ms)(milliseconds to wait=u32 ?) -> ()  [unwired: 1 out]
    }
    "Capture Complete" <- bool ? ("Capture Complete")
  }
  n65 = call "PicoScope6000aClose.vi"("error in (no error)"=w5, "handle in"=w6) -> ()  [unwired: 8 in, 2 out]
